vi "VI-Fix Label.vi"(0 "GObject in":refnum<vi>, 11 "error in (no error)":errorcluster) -> (4 "GObject out":refnum<vi>, 15 "error out":errorcluster)   [LabVIEW 2015]
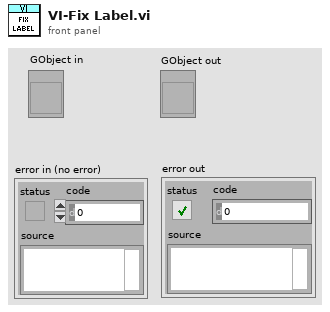
[diagram p1: front panel]
types:
  T1 = typedef "LVRectTypeDef.ctl" = cluster{"Left":i16, "Top":i16, "Right":i16, "Bottom":i16}
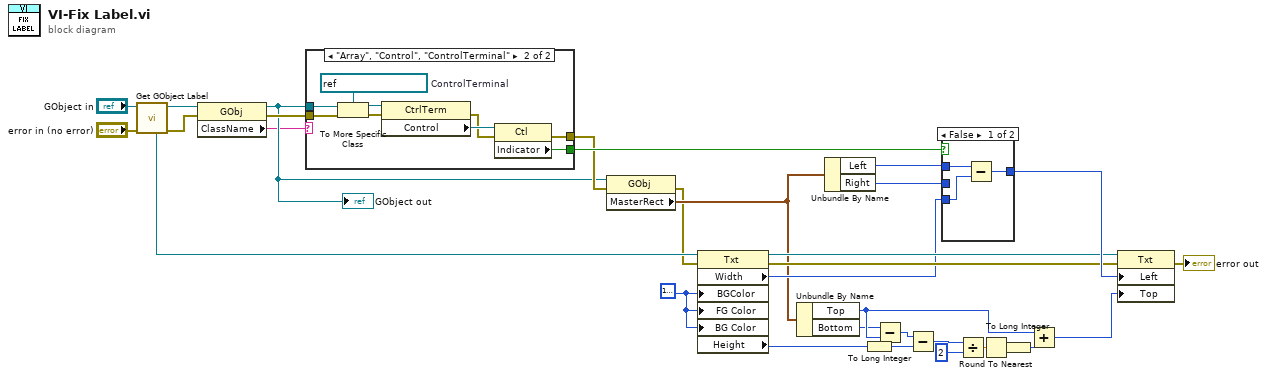
[diagram p0: block diagram]
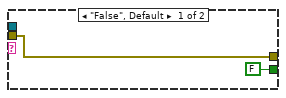
[diagram p2: hidden frame]
diagram:
  w22 = u32 16777216
  n1 = call <vilib>:"Get GObject Label.vi"("error in (no error)"="error in (no error)", "GObject"="GObject in") -> ("error out"=w5:errorcluster, "dup GObject"=w4:refnum<vi>, "Label Reference"=w31:refnum<vi>)  [unwired: 5 in, 2 out]
  n2 = property class="GObj"(reference=w4, error in=w5) -> (reference out=w2:refnum<vi>, error out=w3:errorcluster, "ClassName"=w1:string)
  "GObject out" <- w2
  n3 = case shown="\"Array\", \"Control\", \"ControlTerminal\"" w1 {
    tunnel: [FALSE ("Indicator") w37] -> w26
    tunnel: [w33 w36] -> w7
    tunnel: w3 -> [w33 w35]
    tunnel: w2 -> [_ w34]
    frame "False", Default {
    }
    frame "Array", "Control", "ControlTerminal" {
      w42 = refnum<vi> refnum  # ControlTerminal
      n4 = To More Specific Class(target class=w42, reference=w34, error in=w35) -> (specific class reference=w41:refnum<vi>, error out=w39:errorcluster)
      n5 = property class="CtrlTerm"(reference=w41, error in=w39) -> (error out=w38:errorcluster, "Control"=w40:refnum<vi>)  [unwired: 1 out]
      n6 = property class="Ctl"(reference=w40, error in=w38) -> (error out=w36:errorcluster, "Indicator"=w37:bool)  [unwired: 1 out]
    }
  }
  n7 = property class="GObj"(reference=w2, error in=w7) -> (error out=w6:errorcluster, "MasterRect"=w18:T1)  [unwired: 1 out]
  n8 = property class="Txt"(reference=w31, error in=w6, "BGColor"=w22, "FG Color"=w22, "BG Color"=w22) -> (reference out=w24:refnum<vi>, error out=w23:errorcluster, "Width"=w21:u32, "Height"=w30:u32)
  n9 = Unbundle By Name(w18) -> ("Top"=w16:i16, "Bottom"=w15:i16)
  n10 = Unbundle By Name(w18) -> ("Left"=w19:i16, "Right"=w20:i16)
  n11 = To Long Integer(number=w30) -> (32bit integer=w13:i32)
  n12 = Subtract(x=w15, y=w16) -> (x-y=w17:i16)
  n13 = Subtract(x=w17, y=w13) -> (x-y=w29:i32)
  n14 = case shown="False" w26 {
    tunnel: w19 -> [w44 _]
    tunnel: w20 -> [_ w46]
    tunnel: [w45 w46] -> w25
    tunnel: w21 -> [w43 _]
    frame False {
      n15 = Subtract(x=w44, y=w43) -> (x-y=w45:u32)
    }
    frame True {
    }
  }
  n16 = Divide(x=w29, y=2) -> (x/y=w27:dbl)
  n17 = Round To Nearest(number=w27) -> (nearest integer value=w12:dbl)
  n18 = To Long Integer(number=w12) -> (32bit integer=w11:i32)
  n19 = Add(x=w16, y=w11) -> (x+y=w14:i32)
  n20 = property class="Txt"(reference=w24, error in=w23, "Left"=w25, "Top"=w14) -> (error out=→"error out":errorcluster)  [unwired: 1 out]
